vi "Fit.vi"(7 "Type X":T1(ring), 8 "error in (no error)":errorcluster caption="entrée d'erreur (pas d'erreur)", 9 "y":string[][](array[string]), 10 "X":string[][](array[string]), 11 "StandardScaler.lvclass":refnum<class "StandardScaler.lvclass">) -> (0 "error out":errorcluster caption="sortie d'erreur", 2 "String Data":string, 3 "StandardScaler.lvclass":refnum<class "StandardScaler.lvclass">)   [LabVIEW 2020, in "StandardScaler.lvclass"]
doc: "Compute the mean and std to be used for later scaling.\n\n Returns : \n\n- String OK"
uses:
  StandardScaler.lvclass
  StandardScaler.lvclass/StandardScaler.ctl
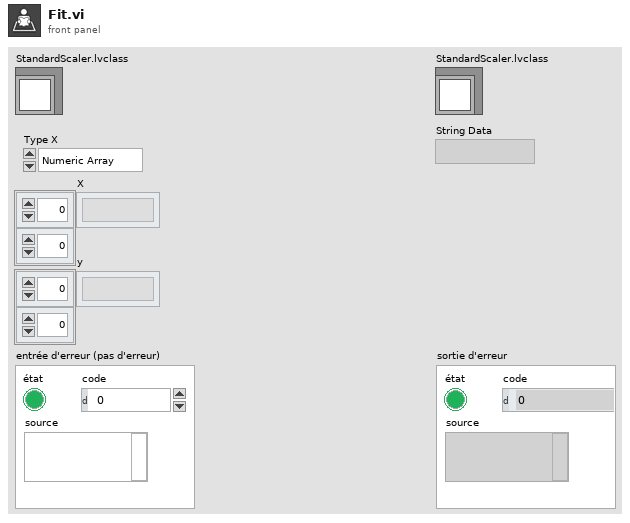
[diagram p1: front panel]
types:
  T1 = enum16{"Numeric Array", "String Array", "Sparse"}
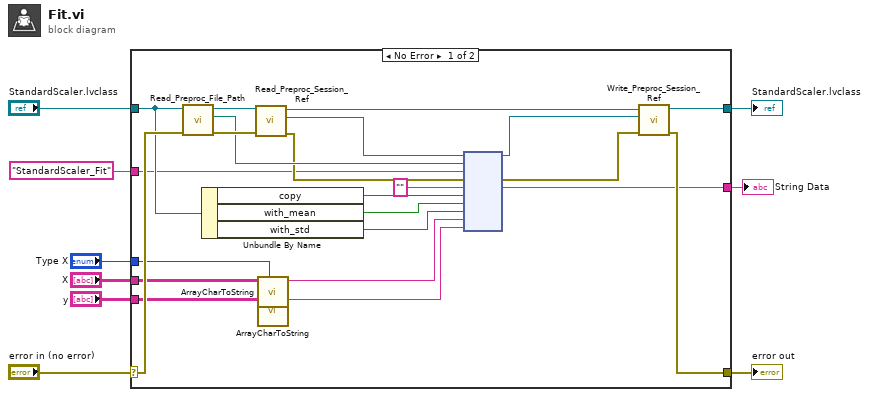
[diagram p0: block diagram]
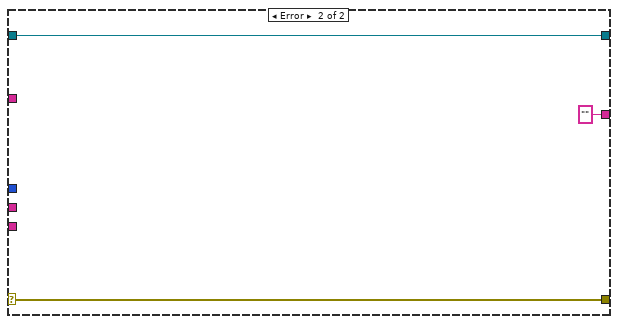
[diagram p2: hidden frame]
diagram:
  n1 = case shown="No Error" "error in (no error)" {
    selector: "error in (no error)" -> [w19 w35]
    tunnel: [w18 w35] -> w8
    tunnel: [w20 w34] -> w6
    tunnel: "StandardScaler.lvclass" -> [w17 w34]
    tunnel: "StandardScaler_Fit" ("Fonction") -> [w16 _]
    tunnel: [w15 ""] -> w4
    tunnel: "X" -> [w14 _]
    tunnel: "y" -> [w13 _]
    tunnel: "Type X" -> [w10 _]
    frame No Error {
      n2 = call-dynamic "Read_Preproc_File_Path.vi"("error in (no error)"=w19, "Python in"=w17) -> ("error out"=w31:errorcluster, "File_Path"=w28:path, "Python out"=w32:refnum<class "StandardScaler.lvclass">)  [unwired: 7 in]
      n3 = Unbundle By Name(w17) -> ("copy"=w23:bool, "with_mean"=w22:bool, "with_std"=w21:bool)
      n4 = call-dynamic "Read_Preproc_Session_Ref.vi"("error in (no error)"=w31, "Python in"=w32) -> ("error out"=w27:errorcluster, "Session_ref"=w29:refnum<k35>, "Python out"=w30:refnum<class "StandardScaler.lvclass">)  [unwired: 7 in]
      n5 = call "ArrayCharToString.vi"("Type"=w10, "TAB"=w14) -> ("Instruction"=w11:string)  [unwired: 9 in]
      n6 = call "ArrayCharToString.vi"("TAB"=w13) -> ("Instruction"=w12:string)  [unwired: 10 in]
      n7 = node(w29, w28, w16, w27, "", w23, w22, w21, w11, w12) -> (w25:refnum<k35>, w26:errorcluster, w15:string)  [unwired: 5 in, 2 out]
      n8 = call-dynamic "Write_Preproc_Session_Ref.vi"("error in (no error)"=w26, "Session_ref"=w25, "Python in"=w30) -> ("error out"=w18:errorcluster, "Python out"=w20:refnum<class "StandardScaler.lvclass">)  [unwired: 7 in]
    }
    frame Error {
    }
  }
  "error out" <- w8
  "StandardScaler.lvclass" <- w6
  "String Data" <- w4
